vi "Get Heartbeat Checker Execution State.vi"(8 "Error In":errorcluster, 11 "reference in":refnum<class "Network Mangement.lvclass">) -> (0 "Error Out":errorcluster, 2 "Exec.State":T1(ring), 3 "reference out":refnum<class "Network Mangement.lvclass">)   [LabVIEW 2024, in "CANopen Master.lvlib" / "Network Mangement.lvclass"]
uses:
  Network Mangement.lvclass
  Network Mangement.lvclass/Network Mangement.ctl
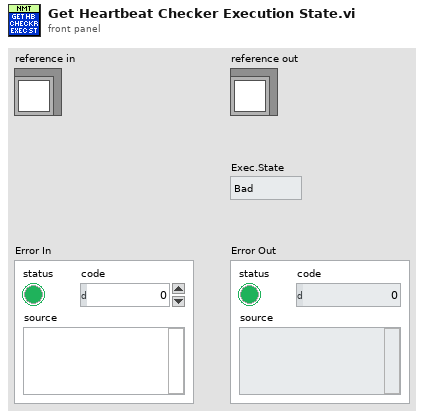
[diagram p1: front panel]
types:
  T1 = enum32{"Bad", "Idle", "Run top level", "Running"}
  T2 = typedef "CANopen Master.lvlib/Network Mangement.lvclass/ObjectAttributes.ctl" = cluster{"Nodes":map{u8, u8}, "Heartbeats":map{u8, cluster{"Period":u16, "Timeout":u16, "Last Beat":timestamp}}, "Events":cluster{"Stop Heartbeat Checker":refnum<user-event>, "Heartbeat Timeout":refnum<user-event>, "Heartbeat Checker Error":refnum<user-event>}, "Heartbeat Checker":refnum<vi>}
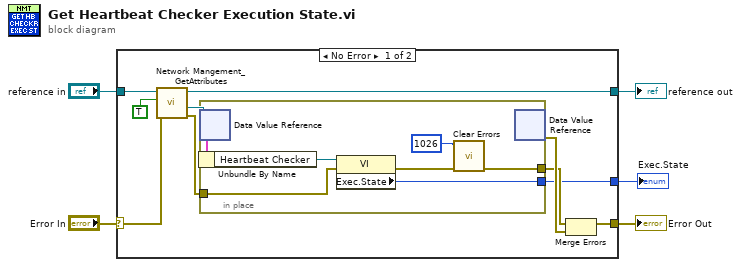
[diagram p0: block diagram]
diagram:
  n1 = case shown="No Error" "Error In" {
    selector: "Error In" -> [w15 w24]
    tunnel: [w14 w24] -> w4
    tunnel: [w11 w23] -> w2
    tunnel: "reference in" -> [w12 w23]
    tunnel: [w6 _] -> w1
    frame No Error {
      n2 = call "Network Mangement_GetAttributes.vi"("Error In"=w15, "OnlyGetDvrReference(False)"=TRUE, "reference in"=w12) -> ("Error Out"=w8:errorcluster, "DataRef"=w9:refnum<data-value>, "reference out"=w11:refnum<class "Network Mangement.lvclass">)  [unwired: 5 in, 1 out]
      n3 = in-place {
        in-place-border: w8 -> [w20]
        in-place-border: [w17] -> w7
        in-place-border: [w16] -> w6
        n4 = in-place-dvr #1(w9) -> (w21:T2)  [unwired: 1 out]
        n5 = Unbundle By Name(w21) -> ("Heartbeat Checker"=w22:refnum<vi>)
        n6 = property class="VI"(reference=w22, error in=w20) -> (error out=w19:errorcluster, "Exec.State"=w16:T1)  [unwired: 1 out]
        n7 = call <vilib>:"Clear Errors.vi"("error in (no error)"=w19, "specific error code to clear (0: all)"=1026) -> ("error out"=w17:errorcluster)  [unwired: 4 in, 1 out]
        n8 = in-place-dvr #1() -> (w13:errorcluster)  [unwired: 1 in, 1 out]
      }
      n9 = Merge Errors(w7, w13) -> (w14:errorcluster)
    }
    frame Error {
    }
  }
  "Error Out" <- w4
  "reference out" <- w2
  "Exec.State" <- w1
